vi "TC to PGSQL.vi"(8 "error in (no error)":errorcluster, 11 "TC Cluster":T1) -> (0 "error out":errorcluster)   [LabVIEW 2013]
uses:
  Typedefs/TC-cluster.ctl
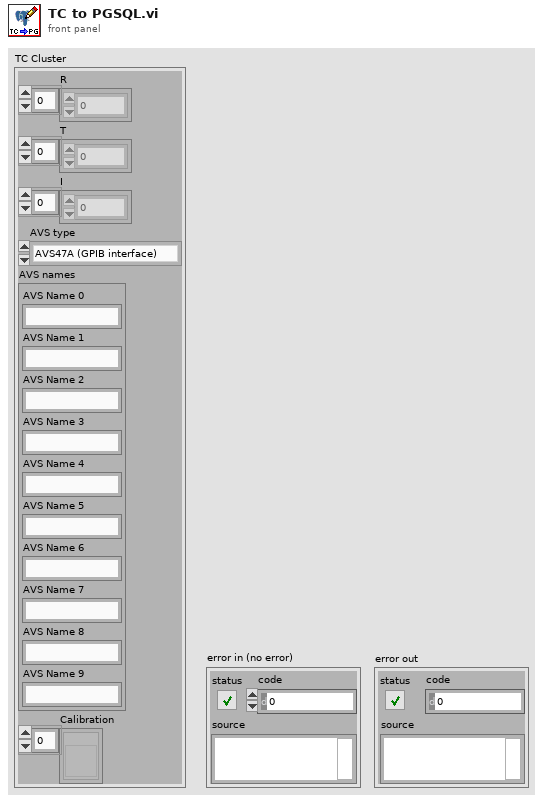
[diagram p1: front panel]
types:
  T1 = typedef "TC-cluster.ctl" = cluster{"R":dbl[], "T":dbl[], "I":dbl[], "AVS type":enum16{"AVS47A (GPIB interface)", "AVS47B (RS232 interface)", "AVS48", "AVS Emulation", "Impedance Bridge", "Disabled"}, "AVS names":cluster{"AVS Name 0":string, "AVS Name 1":string, "AVS Name 2":string, "AVS Name 3":string, "AVS Name 4":string, "AVS Name 5":string, "AVS Name 6":string, "AVS Name 7":string, "AVS Name 8":string, "AVS Name 9":string}, "Calibration":refnum<vi>[]}
  T2 = enum16{"AVS47A (GPIB interface)", "AVS47B (RS232 interface)", "AVS48", "AVS Emulation", "Impedance Bridge", "Disabled"}
  T3 = cluster{"AVS Name 0":string, "AVS Name 1":string, "AVS Name 2":string, "AVS Name 3":string, "AVS Name 4":string, "AVS Name 5":string, "AVS Name 6":string, "AVS Name 7":string, "AVS Name 8":string, "AVS Name 9":string}
  T4 = enum16{"CF", "CF_Z_Bridge", "MNK", "MNK_Z_Bridge"}
  T5 = cluster{"[0]":string, "[1]":string, "[2]":string, "[3]":string, "[4]":string, "[5]":string, "[6]":string, "[7]":string, "[8]":string, "[9]":string}
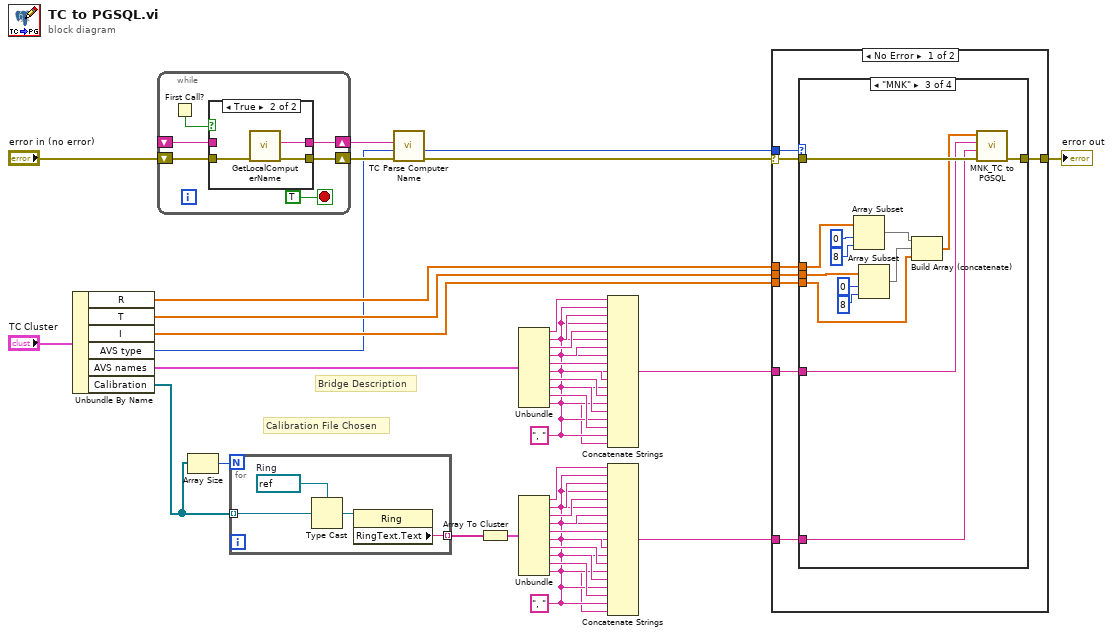
[diagram p0: block diagram]
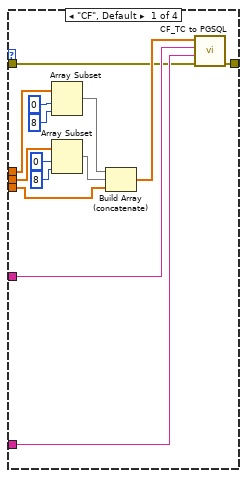
[diagram p3: hidden frame]
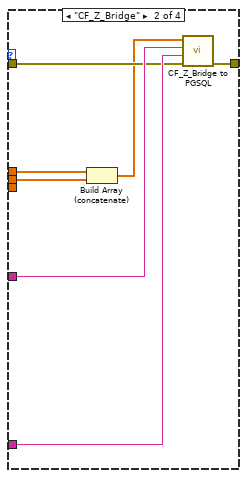
[diagram p4: hidden frame]
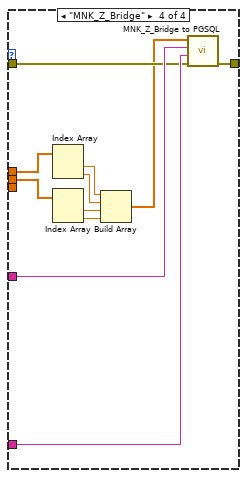
[diagram p5: hidden frame]
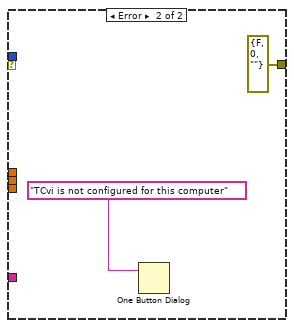
[diagram p6: hidden frame]
diagram:
  w17 = ", " ("string")
  w31 = ", " ("string")
  # "Bridge Description"
  # "Calibration File Chosen"
  n1 = Unbundle By Name("TC Cluster") -> ("R"=w8:dbl[], "T"=w7:dbl[], "I"=w6:dbl[], "AVS type"=w3:T2, "AVS names"=w5:T3, "Calibration"=w4:refnum<vi>[])
  n2 = while {
    shift-right: [w45] -> w11
    shift-left: "error in (no error)" -> [w42]
    shift-right: [w46] -> w2
    shift-left: _ -> [w41]
    stop <- TRUE stop-if-true
    n3 = First Call?() -> (First Call?: T/F=w44:bool)
    n4 = case shown="True" w44 {
      tunnel: [w48 w51] -> w46
      tunnel: [w47 w50] -> w45
      tunnel: w42 -> [w47 w49]
      tunnel: w41 -> [w48 _]
      frame False {
      }
      frame True {
        n5 = call "GetLocalComputerName.vi"("error in (no error)"=w49) -> ("error out"=w50:errorcluster, "Name"=w51:string)  [unwired: 8 in, 1 out]
      }
    }
  }
  n6 = Array Size(array=w4) -> (size(s)=w28:i32)
  n7 = for {
    N: w28 -> [_]
    tunnel: w4 -> [w55] mode=indexing
    tunnel: [w52] -> w27 mode=indexing
    w54 = refnum<vi> refnum  # Ring
    n8 = Type Cast(type=w54, x=w55) -> (*(type *) &x=w53:refnum<vi>)
    n9 = property class="Ring"(reference=w53) -> ("RingText.Text"=w52:string)  [unwired: 1 in, 2 out]
  }
  n10 = call "TC Parse Computer Name.vi"("error in (no error)"=w11, "AVS type"=w3, "computer name"=w2) -> ("error out"=w12:errorcluster, "AVS Type"=w13:T4)  [unwired: 7 in]
  n11 = Array To Cluster(array=w27) -> (cluster=w15:T5)
  n12 = Unbundle(w5) -> ("AVS Name 0"=w40:string, "AVS Name 1"=w39:string, "AVS Name 2"=w38:string, "AVS Name 3"=w37:string, "AVS Name 4"=w36:string, "AVS Name 5"=w35:string, "AVS Name 6"=w34:string, "AVS Name 7"=w33:string, "AVS Name 8"=w32:string, "AVS Name 9"=w30:string)
  n13 = Unbundle(w15) -> ("[0]"=w26:string, "[1]"=w25:string, "[2]"=w24:string, "[3]"=w23:string, "[4]"=w22:string, "[5]"=w21:string, "[6]"=w20:string, "[7]"=w19:string, "[8]"=w18:string, "[9]"=w16:string)
  n14 = Concatenate Strings(w40, w31, w39, w31, w38, w31, w37, w31, w36, w31, w35, w31, w34, w31, w33, w31, w32, w31, w30) -> (w29:string)
  n15 = Concatenate Strings(w26, w17, w25, w17, w24, w17, w23, w17, w22, w17, w21, w17, w20, w17, w19, w17, w18, w17, w16) -> (w14:string)
  n16 = case shown="No Error" w12 {
    selector: w12 -> [w57 _]
    tunnel: w29 -> [w63 _]
    tunnel: w14 -> [w62 _]
    tunnel: w13 -> [w61 _]
    tunnel: w8 -> [w60 _]
    tunnel: w7 -> [w59 _]
    tunnel: w6 -> [w58 _]
    tunnel: [w56 errorcluster {"status"=FALSE, "code"=0, "source"=""} ("error out")] -> w1
    frame No Error {
      n17 = case shown="\"MNK\"" w61 {
        tunnel: w60 -> [w66 w84 w97 w101]
        tunnel: w59 -> [w69 w83 w96 w100]
        tunnel: w58 -> [w70 _ w86 _]
        tunnel: w63 -> [w77 w82 w91 w105]
        tunnel: w62 -> [w76 w81 w92 w104]
        tunnel: w57 -> [w64 w80 w94 w103]
        tunnel: [w65 w79 w93 w102] -> w56
        frame "CF", Default {
          n18 = Array Subset(array=w66, index=0, length=8) -> (w68:dbl[])
          n19 = Array Subset(array=w69, index=0, length=8) -> (w67:dbl[])
          n20 = Build Array (concatenate)(w68, w67, w70) -> (w75:dbl[])
          n21 = call "CF_TC to PGSQL.vi"("error in (no error)"=w64, "calibration string"=w76, "description string"=w77, "dbl"=w75) -> ("error out"=w65:errorcluster)  [unwired: 7 in]
        }
        frame "CF_Z_Bridge" {
          n22 = Build Array (concatenate)(w84, w83) -> (w78:dbl[])
          n23 = call "CF_Z_Bridge to PGSQL.vi"("error in (no error)"=w80, "calibration string"=w81, "description string"=w82, "dbl"=w78) -> ("error out"=w79:errorcluster)  [unwired: 7 in]
        }
        frame "MNK" {
          n24 = Array Subset(array=w97, index=0, length=8) -> (w87:dbl[])
          n25 = Array Subset(array=w96, index=0, length=8) -> (w95:dbl[])
          n26 = Build Array (concatenate)(w87, w95, w86) -> (w85:dbl[])
          n27 = call "MNK_TC to PGSQL.vi"("error in (no error)"=w94, "calibration string"=w92, "description string"=w91, "dbl"=w85) -> ("error out"=w93:errorcluster)  [unwired: 7 in]
        }
        frame "MNK_Z_Bridge" {
          n28 = Index Array(array=w101) -> (element #1=w109:dbl, element #2=w108:dbl)  [unwired: 2 in]
          n29 = Index Array(array=w100) -> (element #1=w107:dbl, element #2=w106:dbl)  [unwired: 2 in]
          n30 = Build Array(w109, w108, w107, w106) -> (w99:dbl[])
          n31 = call "MNK_Z_Bridge to PGSQL.vi"("error in (no error)"=w103, "calibration string"=w104, "description string"=w105, "dbl"=w99) -> ("error out"=w102:errorcluster)  [unwired: 7 in]
        }
      }
    }
    frame Error {
      n32 = One Button Dialog(message="TCvi is not configured for this computer" ("URL")) -> ()  [unwired: 1 in, 1 out]
    }
  }
  "error out" <- w1
